vi "timeout.vi"(0 "Time Target (s)":dbl=3.0 caption="Zielzeit (s)", 2 "Reset":bool caption="Zurücksetzen", 3 "Auto Reset":bool=TRUE caption="Autom. zurücksetzen", 5 "error in (no error)":errorcluster caption="Fehler (Eingang, kein Fehler)", 8 "Set Start Time (s)":dbl caption="Startzeit festlegen (s)") -> (11 "Get Start Time (s)":dbl caption="Startzeit lesen (s)", 13 "Start Time Text":string caption="Startzeit (Text)", 14 "Present (s)":dbl caption="Aktuell (s)", 15 "Present Text":string caption="Aktuell (Text)", 16 "Elapsed Time (s)":dbl caption="Verstrichene Zeit (s)", 17 "Time has Elapsed":bool caption="Zeit ist verstrichen", 18 "Elapsed Time Text":string caption="Verstrichene Zeit (Text)", 19 "error out":errorcluster caption="Fehler (Ausgang)")   [LabVIEW 2012]
doc: "Zeigt die seit Zählbeginn vergangene Zeit an.\n--------------------\n\nDieses Express-VI ist wie folgt konfiguriert:\n\nZielzeit: 3 s\nAutom. zurücksetzen: Ein"
panel:
  # "Zurücksetzen, sobald Zeit abgelaufen ist."
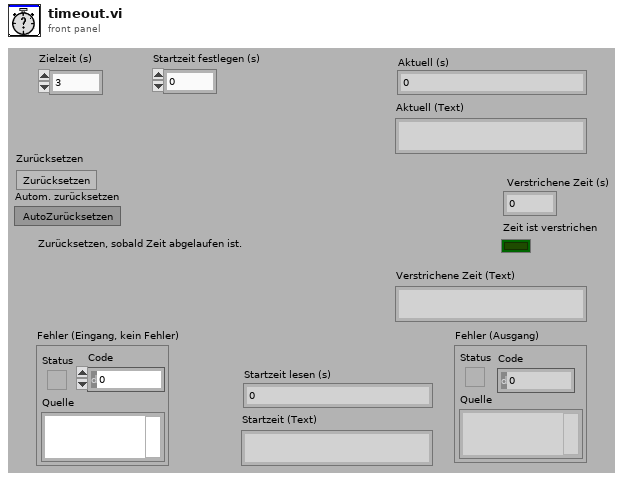
[diagram p1: front panel]
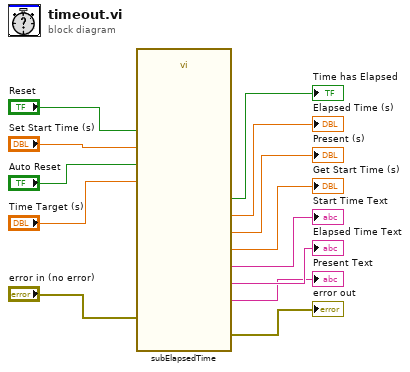
[diagram p0: block diagram]
diagram:
  n1 = call <vilib>:"subElapsedTime.vi"("Reset"="Reset", "Elapsed Time Target"="Time Target (s)", "Set Start Time"="Set Start Time (s)", "Auto Reset"="Auto Reset", "error in (no error)"="error in (no error)") -> ("Elapsed TimeText"=→"Elapsed Time Text":string, "Present Text"=→"Present Text":string, "Start Time Text"=→"Start Time Text":string, "Time has Elapsed"=→"Time has Elapsed":bool, "Elapsed Time"=→"Elapsed Time (s)":dbl, "Present"=→"Present (s)":dbl, "Get Start Time"=→"Get Start Time (s)":dbl, "error out"=→"error out":errorcluster)  [unwired: 7 in]
